vi "Step SSI.vi"(10 "Step Deployment State":T3, 11 "Robot Controls":T4) -> (3 "Step Actuator Values Out":T1)   [LabVIEW 2014]
uses:
  Robot Commands.ctl
  Step Deployment SS State.ctl
  Step Deployment Actuator Values.ctl
  <vilib>/Rock Robotics/WPI/Solenoid/WPI_SolenoidValue.ctl
panel:
  # "Field Centric"
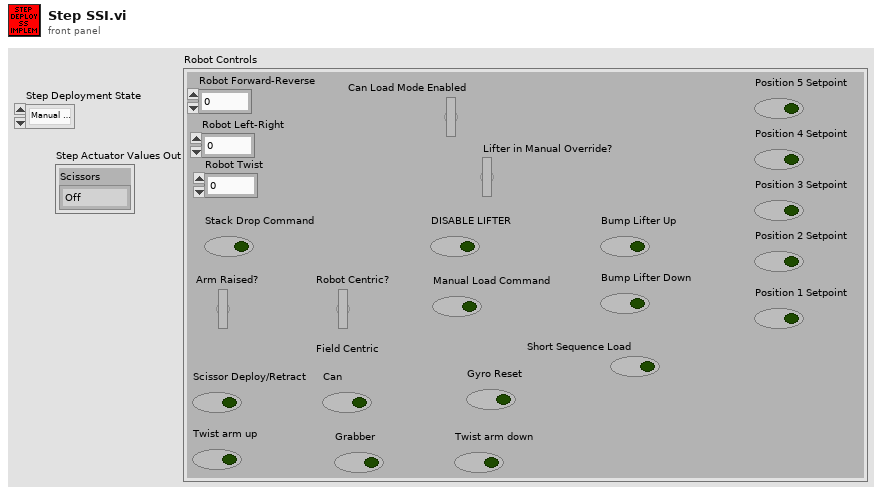
[diagram p1: front panel]
types:
  T1 = typedef "Step Deployment Actuator Values.ctl" = cluster{"Scissors":T2}
  T2 = typedef "WPI_SolenoidValue.ctl" = enum16{"Off", "On", "Forward", "Reverse"}
  T3 = typedef "Step Deployment SS State.ctl" = enum16{"Manual Override", "Disabled"}
  T4 = typedef "Robot Commands.ctl" = cluster{"Robot Forward-Reverse":dbl, "Robot Left-Right":dbl, "Robot Twist":dbl, "Can Load Mode Enabled":bool, "Lifter in Manual Override?":bool, "Stack Drop Command":bool, "Arm Raised?":bool, "DISABLE LIFTER":bool, "Position 1 Setpoint":bool, "Position 2 Setpoint":bool, "Position 3 Setpoint":bool, "Position 4 Setpoint":bool, "Position 5 Setpoint":bool, "Bump Lifter Down":bool, "Bump Lifter Up":bool, "Manual Load Command":bool, "Robot Centric?":bool, "Scissor Deploy/Retract":bool, "Grabber":bool, "Can":bool, "Twist arm up":bool, "Gyro Reset":bool, "Twist arm down":bool, "Short Sequence Load":bool}
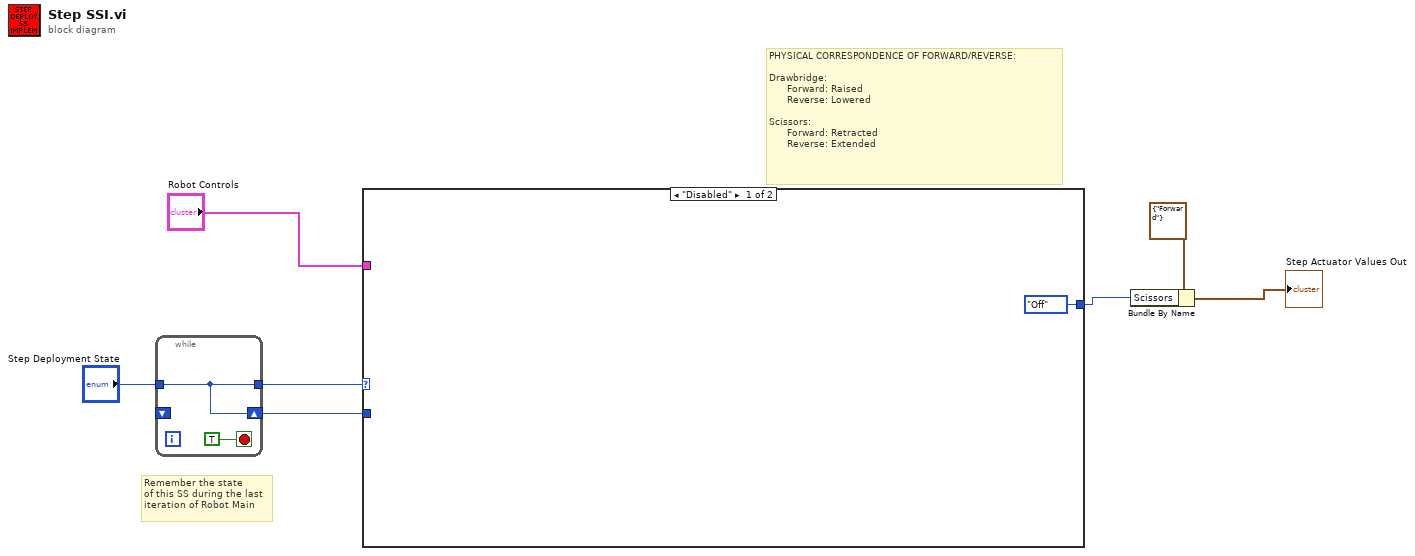
[diagram p0: block diagram]
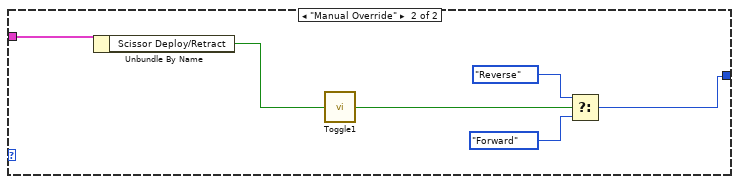
[diagram p2: hidden frame]
diagram:
  # "Remember the state\nof this SS during the last\niteration of Robot Main"
  # "PHYSICAL CORRESPONDENCE OF FORWARD/REVERSE:\n\nDrawbridge:\n      Forward: Raised\n      Reverse: Lowered\n\nScissors:\n      Forward: Retracted\n      Reverse: Extended"
  n1 = while {
    tunnel: "Step Deployment State" -> [w8]
    tunnel: [w8] -> w2
    shift-right: [w8] -> w1
    shift-left: _ -> [_]
    stop <- TRUE stop-if-true
  }
  n2 = case shown="\"Disabled\"" w2 {
    tunnel: "Robot Controls" -> [_ w16]
    tunnel: [WPI_SolenoidValue."Off" ("Scissors") w13] -> w6
    tunnel: w1 -> [_ _]
    frame "Disabled" {
    }
    frame "Manual Override" {
      n3 = Unbundle By Name(w16) -> ("Scissor Deploy/Retract"=w12:bool)
      n4 = call "Toggle1.vi"("Boolean"=w12) -> ("Driver Switch 2"=w11:bool)
      n5 = Select(t=WPI_SolenoidValue."Reverse" ("Scissors"), s=w11, f=WPI_SolenoidValue."Forward" ("Scissors")) -> (s? t:f=w13:T2)
    }
  }
  n6 = Bundle By Name(cluster=T1 {"Scissors"=enum."Forward"}, "Scissors"=w6) -> (→"Step Actuator Values Out":T1)
